vi "Drive Straight Arcade.vi"(11 "Angle robot facing":dbl) -> (3 "Arcade drive x":dbl)   [LabVIEW 2017]
uses:
  <vilib>/addons/control/pid/pid.llb/PID (DBL).vi
  <vilib>/addons/control/pid/NI_PID_pid.lvlib
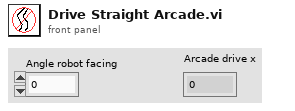
[diagram p1: front panel]
types:
  T1 = cluster{"proportional gain (Kc)":dbl, "integral time (Ti, min)":dbl, "derivative time (Td, min)":dbl}
  T2 = typedef "WPI_GyroDevRef.ctl" = cluster{"DevStatus":errorcluster, "Analog Channel":T3, "Gain (VoltsPerDegree/Second)":dbl, "Gyro Type":enum16{"Analog", "XRS450"}, "Handle":i32, "SPI Bus":T4, "Device Found":bool, "Sample Rate":dbl, "Calibrate On Open":bool, "Offset":dbl}
  T3 = typedef "FPGA_AIChannel.ctl" = enum8{"AI 0", "AI 1", "AI 2", "AI 3", "AI MXP 0", "AI MXP 1", "AI MXP 2", "AI MXP 3", "Invalid"}
  T4 = typedef "spi_bus.ctl" = enum16{"SPI On-Board, CS0", "SPI On-Board, CS1", "SPI On-Board, CS2", "SPI On-Board, CS3", "SPI MXP", "Invalid"}
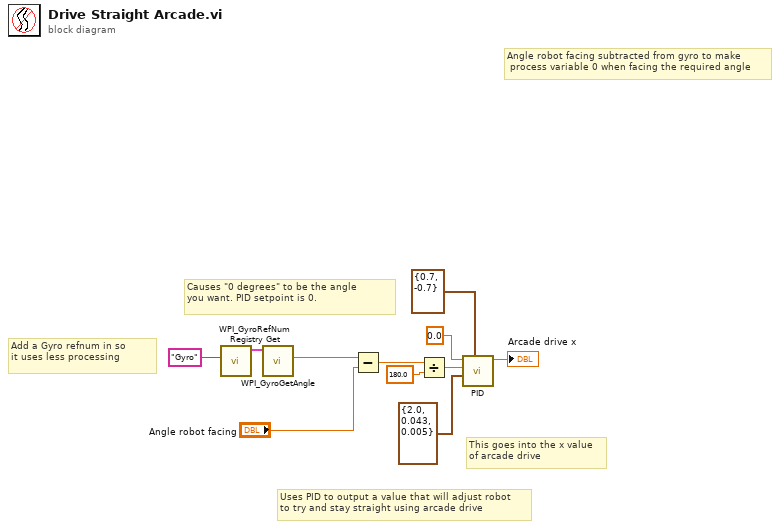
[diagram p0: block diagram]
diagram:
  # "Add a Gyro refnum in so\nit uses less processing"
  # "Causes \"0 degrees\" to be the angle\nyou want. PID setpoint is 0."
  # "This goes into the x value \nof arcade drive"
  # "Angle robot facing subtracted from gyro to make\n process variable 0 when facing the required angle"
  # "Uses PID to output a value that will adjust robot\nto try and stay straight using arcade drive"
  n1 = call <vilib>:"WPI_GyroRefNum Registry Get.vi"("refnum name"="Gyro") -> ("GyroDevRef"=w6:T2)  [unwired: 9 in, 1 out]
  n2 = call <vilib>:"WPI_GyroGetAngle.vi"("GyroDevRef"=w6) -> ("Angle"=w1:dbl)  [unwired: 6 in, 4 out]
  n3 = Subtract(x=w1, y="Angle robot facing") -> (x-y=w10:dbl)
  n4 = Divide(x=w10, y=180.0) -> (x/y=w8:dbl)
  n5 = call-poly <vilib>:"PID.vi"("output range"=cluster{"output high":dbl, "output low":dbl} {"output high"=0.7, "output low"=-0.7}, "PID gains"=T1 {"proportional gain (Kc)"=2.0, "integral time (Ti, min)"=0.043, "derivative time (Td, min)"=0.005} ("Drive straight"), "process variable"=w8, "setpoint"=0.0) -> ("output"=→"Arcade drive x":dbl)  [unwired: 6 in, 1 out]
